vi "Read IL State.vi"(9 "Index":i32=-1, 10 "In Chain":T1=enum."None", 11 "Interlock Chain in":refnum<class "Interlock Chain.lvclass">) -> (2 "State":T2, 3 "Interlock Chain out":refnum<class "Interlock Chain.lvclass">)   [LabVIEW 2015, in "Interlocks.lvlib" / "Interlock Chain.lvclass"]
uses:
  Interlock Chain.lvclass
  Interlock/State Enum.ctl
  Controls/Add IL to -Enumerator.ctl
  Interlock Chain.lvclass/Interlock Chain.ctl
  Interlock/Interlock.lvclass
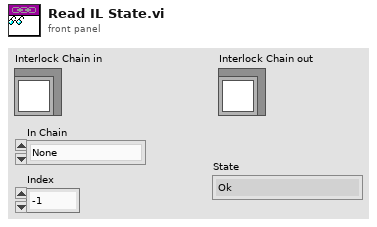
[diagram p1: front panel]
types:
  T1 = typedef "Add IL to -Enumerator.ctl" = enum16{"Deny", "Allow", "None"}
  T2 = typedef "Interlocks.lvlib/Interlock.lvclass/State Enum.ctl" = enum16{"Ok", "Error", "Interlock", "Out of Range", "Is ON", "Is OFF", "Denied", "Not Allowed", "Sample Allow", "Sample Deny"}
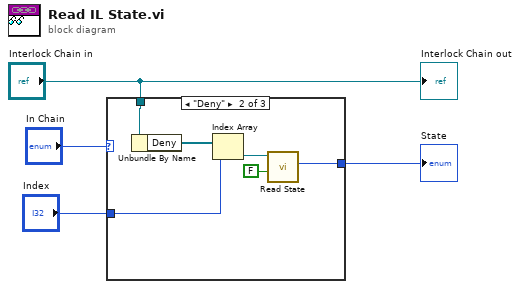
[diagram p0: block diagram]
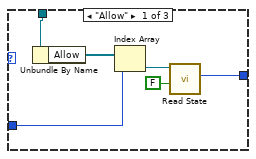
[diagram p2: hidden frame]
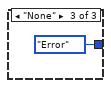
[diagram p3: hidden frame]
diagram:
  n1 = case shown="\"Deny\"" "In Chain" {
    tunnel: "Index" -> [w8 w14 _]
    tunnel: "Interlock Chain in" -> [w10 w16 _]
    tunnel: [w5 w11 State_Enum."Error" ("State")] -> w1
    frame "Allow" {
      n2 = Unbundle By Name(w10) -> ("Allow"=w9:refnum<class "Interlock.lvclass">[])
      n3 = Index Array(array=w9, index=w8) -> (element=w7:refnum<class "Interlock.lvclass">)
      n4 = call "Read State.vi"("String (T)"=FALSE, "Interlock in"=w7) -> ("State"=w5:T2)  [unwired: 7 in, 2 out]
    }
    frame "Deny" {
      n5 = Unbundle By Name(w16) -> ("Deny"=w15:refnum<class "Interlock.lvclass">[])
      n6 = Index Array(array=w15, index=w14) -> (element=w13:refnum<class "Interlock.lvclass">)
      n7 = call "Read State.vi"("String (T)"=FALSE, "Interlock in"=w13) -> ("State"=w11:T2)  [unwired: 7 in, 2 out]
    }
    frame "None" {
    }
  }
  "State" <- w1
  "Interlock Chain out" <- "Interlock Chain in"
